vi "Set NumLock.vi"(8 "error in (no error)":errorcluster, 11 "Numeric in":refnum<class "Numeric.lvclass">) -> (0 "error out":errorcluster, 3 "Keypad out":refnum<class "Keypad.lvclass">)   [LabVIEW 2020, in "Keypad.lvlib" / "Numeric.lvclass"]
uses:
  Numeric.lvclass
  Cursor/Cursor.lvclass
  <vilib>/ni/Actors/State Actor/State Actor/State Actor.lvclass
  Keypad/Keypad.lvclass
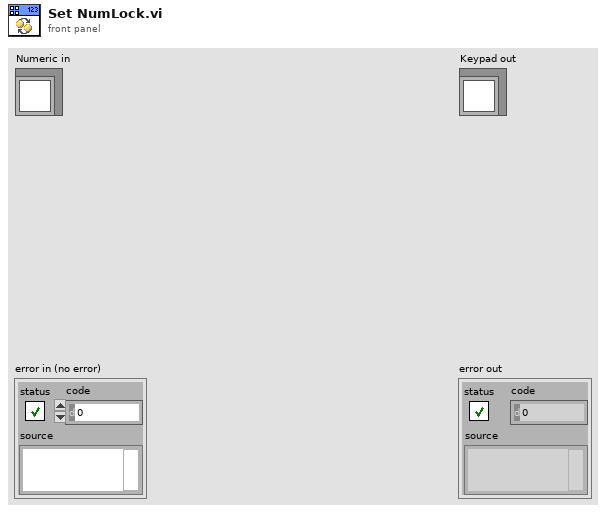
[diagram p1: front panel]
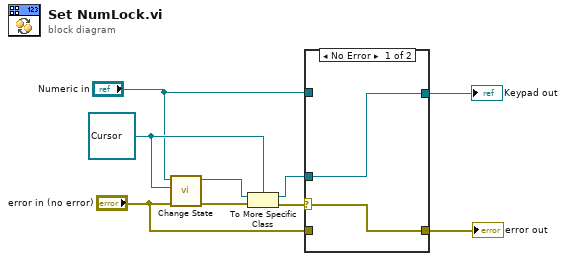
[diagram p0: block diagram]
diagram:
  w7 = refnum<class "Cursor.lvclass"> refnum ("Keypad.lvlib:Cursor.lvclass")
  n1 = call <vilib>:"Change State.vi"("error in (no error)"="error in (no error)", "New State in"=w7, "State in"="Numeric in") -> ("error out"=w8:errorcluster, "State out"=w9:refnum<class "State Actor.lvclass">)  [unwired: 7 in]
  n2 = To More Specific Class(target class=w7, reference=w9, error in=w8) -> (specific class reference=w5:refnum<class "Cursor.lvclass">, error out=w6:errorcluster)
  n3 = case shown="No Error" w6 {
    selector: w6 -> [w10 _]
    tunnel: w5 -> [w11 _]
    tunnel: [w11 w12] -> w4
    tunnel: [w10 w13] -> w3
    tunnel: "error in (no error)" -> [_ w13]
    tunnel: "Numeric in" -> [_ w12]
    frame No Error {
    }
    frame Error {
    }
  }
  "error out" <- w3
  "Keypad out" <- w4
